vi "util_run_subs.vi"(8 "error in (no error)":errorcluster) -> (0 "error out":errorcluster, 3 "interface []":T1[](array[typedef]))   [LabVIEW 2015, in "lv-interface-dom-nre.lvlib"]
uses:
  lv-interface-dom-nre.lvlib
  _controls/interface_refnum.ctl
  lv-interface-sub-common/_controls/interface_selection.ctl
  lv-interface-sub-re/lv-interface-sub-re.lvlib
  lv-interface-sub-common/lv-interface-sub-common.lvlib
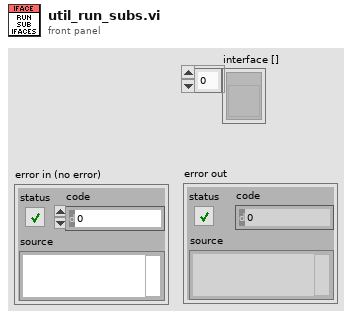
[diagram p1: front panel]
types:
  T1 = typedef "lv-interface-dom-nre.lvlib/interface_refnum.ctl" = refnum<vi>
  T2 = typedef "lv-interface-sub-common.lvlib/interface_selection.ctl" = enum16{"<interface>", "sub_interface_1", "sub_interface_2", "<null>"}
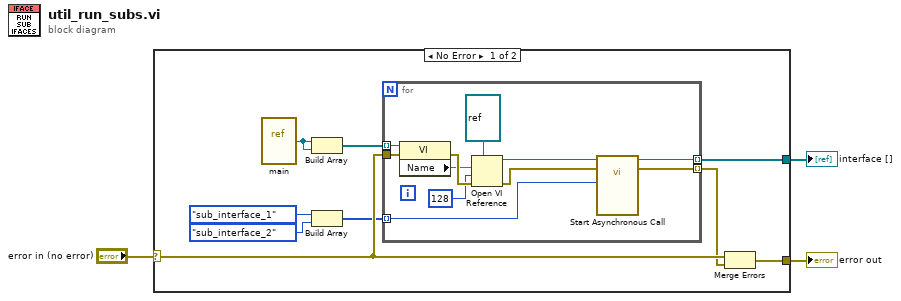
[diagram p0: block diagram]
diagram:
  n1 = case shown="No Error" "error in (no error)" {
    selector: "error in (no error)" -> [w10 w24]
    tunnel: [w12 _] -> w3
    tunnel: [w11 w24] -> w2
    frame No Error {
      n2 = vi-ref "main.vi"() -> (w7:refnum<vi>)
      n3 = Build Array(w7, w7) -> (w8:refnum<vi>[])
      n4 = Build Array(interface_selection."sub_interface_1" ("interface"), interface_selection."sub_interface_2" ("interface")) -> (w4:T2[])
      n5 = for {
        tunnel: [w15] -> w12 mode=indexing
        tunnel: w10 -> [w20]
        tunnel: [w14] -> w9 mode=indexing
        tunnel: w8 -> [w22] mode=indexing
        tunnel: w4 -> [w16] mode=indexing
        n6 = property class="VI"(reference=w22, error in=w20) -> (error out=w23:errorcluster, "Name"=w21:string)  [unwired: 1 out]
        n7 = Open VI Reference(type specifier VI Refnum (for type only)=refnum<vi> refnum, vi path=w21, options=128, error in (no error)=w23) -> (vi reference=w18:refnum<vi>, error out=w17:errorcluster)  [unwired: 2 in]
        n8 = call-by-ref "Start Asynchronous Call"(reference=w18, error in=w17, "interface"=w16) -> (reference out=w15:refnum<vi>, error out=w14:errorcluster)  [unwired: 10 in, 1 out]
      }
      n9 = Merge Errors(w10, w9) -> (w11:errorcluster)
    }
    frame Error {
    }
  }
  "error out" <- w2
  "interface []" <- w3
